vi "Link Status.vi"(5 "Username":string, 6 "Password":string, 7 "Address":string, 8 "Error In":errorcluster) -> (0 "Error Out":errorcluster)   [LabVIEW 2018, in "Tests.lvlib" / "SFTP.lvlib"]
uses:
  SFTP.lvlib
  src/Toolkit/SFTP Attributes/Support/Create from SFTP.vi
  src/Toolkit/SFTP Attributes/Support/Destroy to SFTP.vi
  <vilib>/addons/_JKI Toolkits/Caraya/classes/Test/Test.lvclass
  <vilib>/addons/_JKI Toolkits/Caraya/classes/Assert/Assert.lvclass
  src/Toolkit/SFTP/SFTP.lvclass
  src/Toolkit/SFTP Attributes/SFTP Attributes.lvclass
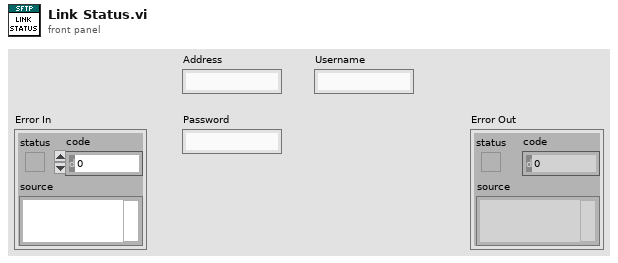
[diagram p1: front panel]
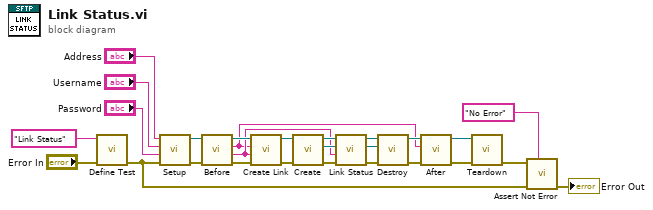
[diagram p0: block diagram]
diagram:
  n1 = call <vilib>:"Define Test.vi"("error in (no error)"="Error In", "Label (VI Title)"="Link Status") -> ("error out"=w23:errorcluster)  [unwired: 9 in]
  n2 = call "Setup.vi"("Error In"=w23, "Password"="Password", "Username"="Username", "Address"="Address") -> ("Error Out"=w11:errorcluster, "Sesssion"=w12:refnum<class "Session.lvclass">)  [unwired: 6 in]
  n3 = call "Before.vi"("Error In"=w11, "Session In"=w12) -> ("Error Out"=w9:errorcluster, "Remote Link Path"=w7:string, "Remote Source Path"=w3:string, "SFTP Out"=w10:refnum<class "SFTP.lvclass">)  [unwired: 6 in]
  n4 = call "Create Link.vi"("Error In"=w9, "Remote Link Path"=w7, "Remote Source Path"=w3, "SFTP In"=w10) -> ("Error Out"=w8:errorcluster, "SFTP Out"=w13:refnum<class "SFTP.lvclass">)  [unwired: 6 in]
  n5 = call-poly "Create.vi"("Error In"=w8, "SFTP In"=w13) -> ("Error Out"=w6:errorcluster, "SFTP Attributes"=w17:refnum<class "SFTP Attributes.lvclass">, "SFTP Out"=w18:refnum<class "SFTP.lvclass">)  [unwired: 7 in]
  n6 = call "Link Status.vi"("Error In"=w6, "Remote Path"=w7, "Attributes In"=w17, "SFTP In"=w18) -> ("Error Out"=w14:errorcluster, "Attributes Out"=w15:refnum<class "SFTP Attributes.lvclass">, "SFTP Out"=w16:refnum<class "SFTP.lvclass">)  [unwired: 5 in]
  n7 = call-poly "Destroy.vi"("Error In"=w14, "SFTP Attributes"=w15, "SFTP In"=w16) -> ("Error Out"=w4:errorcluster, "SFTP Out"=w5:refnum<class "SFTP.lvclass">)  [unwired: 7 in]
  n8 = call "After.vi"("Error In"=w4, "Remote Source Path"=w3, "SFTP In"=w5) -> ("Error Out"=w2:errorcluster, "Session Out"=w1:refnum<class "Session.lvclass">)  [unwired: 7 in]
  n9 = call "Teardown.vi"("Error In"=w2, "Session"=w1) -> ("Error Out"=w19:errorcluster)  [unwired: 9 in]
  n10 = call <vilib>:"Assert Not Error.vi"("Label"="No Error", "error in (no error)"=w23, "Not Error?"=w19) -> ("error out"=→"Error Out":errorcluster)  [unwired: 8 in]
